vi "Read SM1000 positions.vi"(8 "error in (no error)":errorcluster, 11 "HC-Main in":refnum<class "MC-Main.lvclass">) -> (0 "error out":errorcluster, 2 "SM1000 positions":i16[][](array[numeric]), 3 "HC-Main out":refnum<class "MC-Main.lvclass">)   [LabVIEW 2013, in "MaterialCharacterization.lvlib" / "MC-Main.lvclass"]
uses:
  MC-Main.lvclass
  MC-Main.lvclass/MC-Main.ctl
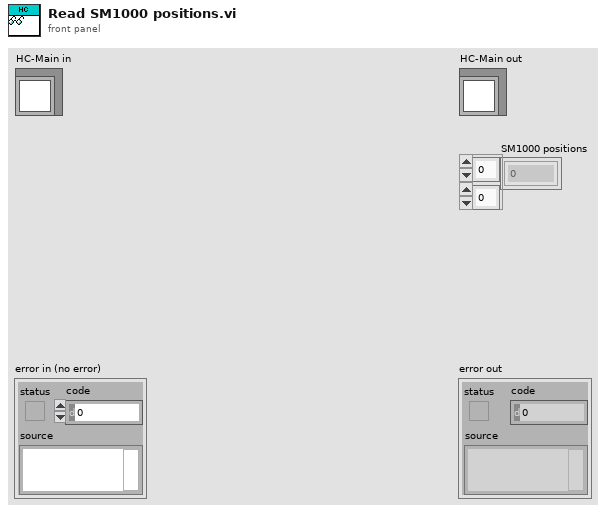
[diagram p1: front panel]
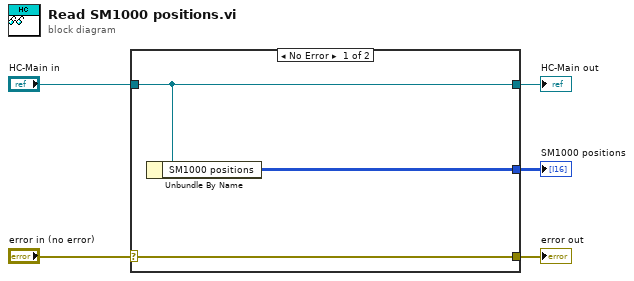
[diagram p0: block diagram]
diagram:
  n1 = case shown="No Error" "error in (no error)" {
    selector: "error in (no error)" -> [w8 w9]
    tunnel: [w8 w9] -> w4
    tunnel: [w7 w10] -> w2
    tunnel: "HC-Main in" -> [w7 w10]
    tunnel: [w6 _] -> w1
    frame No Error {
      n2 = Unbundle By Name(w7) -> ("SM1000 positions"=w6:i16[][])
    }
    frame Error {
    }
  }
  "error out" <- w4
  "HC-Main out" <- w2
  "SM1000 positions" <- w1
